vi "Destroy.vi"(8 "error in (no error)":errorcluster, 11 "Plugin Manager in":refnum<class "CIFLauncher.lvclass">) -> (0 "error out":errorcluster, 3 "Plugin Manager out":refnum<class "CIFLauncher.lvclass">)   [LabVIEW 2021, in "CIFLauncher.lvclass"]
uses:
  CIFLauncher.lvclass
  CIFUtilities/CIFLogs/Typedef/Message Type.ctl
  CIFLauncher.lvclass/CIFLauncher.ctl
  <vilib>/gRPC/LabVIEW gRPC Servicer/ServiceBase/ServiceBase.lvclass
  CIFUtilities/CIFLogs/CIFLogs.lvlib
  typedef/Loaded Plugin Map.ctl
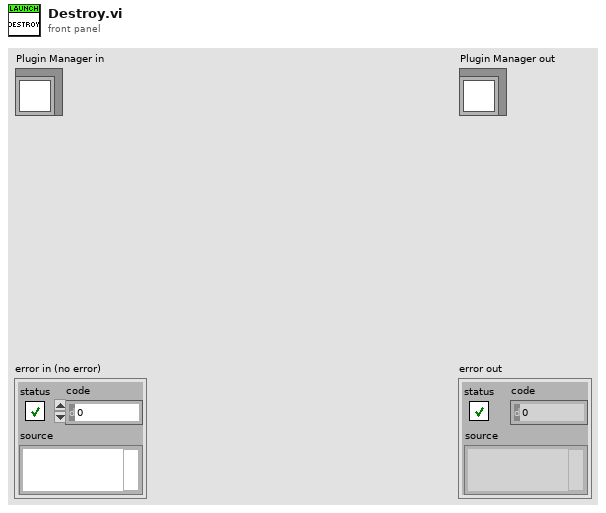
[diagram p1: front panel]
types:
  T1 = typedef "CIFLogs.lvlib/Message Type.ctl" = enum16{"Error", "Information", "Print Terminal", "Configuration"}
  T2 = typedef "CIFLauncher.lvclass/Loaded Plugin Map.ctl" = map{string, refnum<vi>}
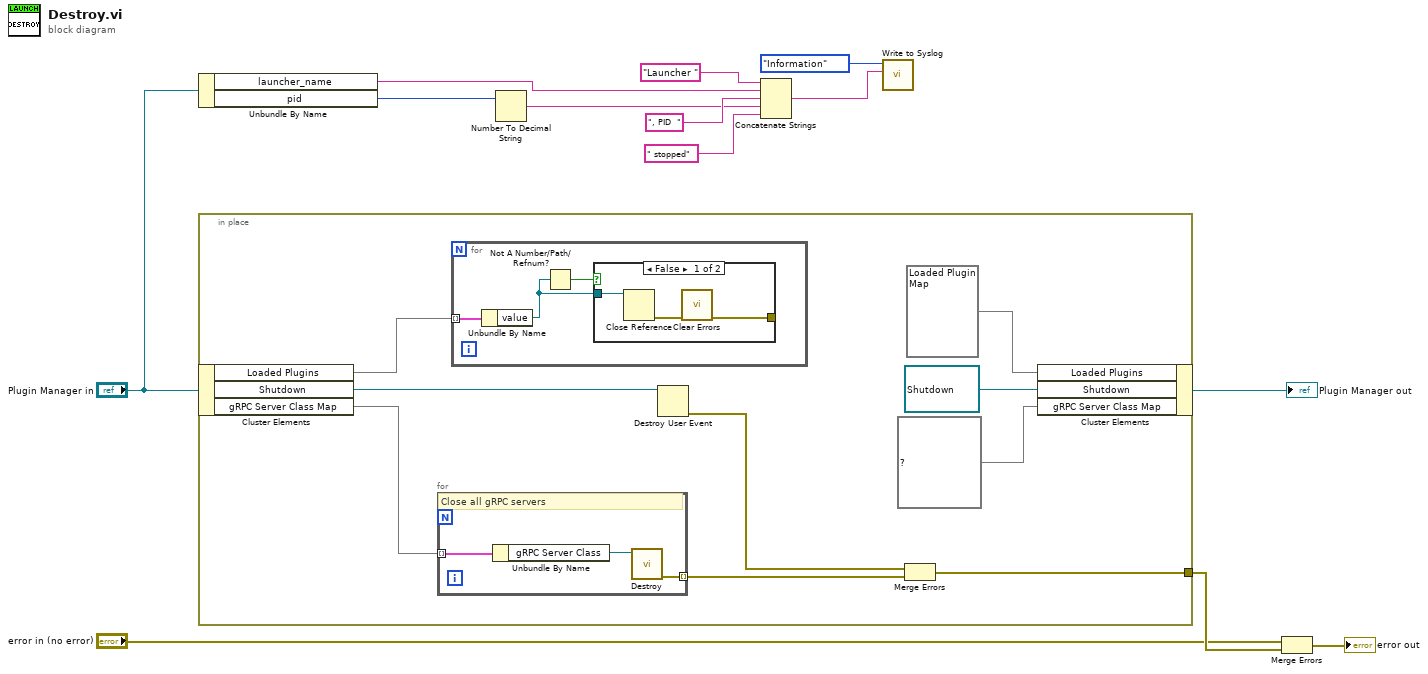
[diagram p0: block diagram]
diagram:
  n1 = Unbundle By Name("Plugin Manager in") -> ("launcher_name"=w3:string, "pid"=w4:u32)
  n2 = in-place {
    in-place-border: [w19] -> w12
    n3 = in-place-cluster #1("Plugin Manager in") -> ("Loaded Plugins"=w15:T2, "Shutdown"=w18:refnum<user-event>, "gRPC Server Class Map"=w22:map{string, refnum<class "ServiceBase.lvclass">})
    n4 = for {
      tunnel: w22 -> [w31] mode=indexing
      tunnel: [w29] -> w20 mode=indexing
      # "Close all gRPC servers"
      n5 = Unbundle By Name(w31) -> ("gRPC Server Class"=w30:refnum<class "ServiceBase.lvclass">)
      n6 = call-dynamic "Destroy.vi"("SignalGeneratorService in"=w30) -> ("error out"=w29:errorcluster)  [unwired: 9 in, 1 out]
    }
    n7 = for {
      tunnel: w15 -> [w24] mode=indexing
      n8 = Unbundle By Name(w24) -> ("value"=w23:refnum<vi>)
      n9 = Not A Number/Path/Refnum?(number/path/refnum=w23) -> (NaN/Path/Refnum?=w25:bool)
      n10 = case shown="False" w25 {
        tunnel: w23 -> [w28 _]
        tunnel: [w26 _] -> _
        frame False {
          n11 = Close Reference(reference=w28) -> (error out=w27:errorcluster)  [unwired: 1 in]
          n12 = call <vilib>:"Clear Errors.vi"("error in (no error)"=w27) -> ("error out"=w26:errorcluster)  [unwired: 5 in, 1 out]
        }
        frame True {
        }
      }
    }
    n13 = Destroy User Event(user event=w18) -> (error out=w17:errorcluster)  [unwired: 1 in]
    n14 = Merge Errors(w17, w20) -> (w19:errorcluster)
    n15 = in-place-cluster #1("Loaded Plugins"=T2 {}, "Shutdown"=refnum<user-event> refnum ("Parallel Events.Shutdown"), "gRPC Server Class Map"=map{string, refnum<class "ServiceBase.lvclass">} {}) -> (→"Plugin Manager out":refnum<class "CIFLauncher.lvclass">)
  }
  n16 = Number To Decimal String(number=w4) -> (decimal integer string=w6:string)  [unwired: 1 in]
  n17 = Concatenate Strings("Launcher " ("message"), w3, ", PID  " ("message"), w6, " stopped" ("message")) -> (w2:string)
  n18 = call "Write to Syslog.vi"("message"=w2, "CIF Message Type"=Message_Type."Information") -> ()  [unwired: 9 in, 1 out]
  n19 = Merge Errors("error in (no error)", w12) -> (→"error out":errorcluster)
